vi "methane method.vi"(7 "pattern":string, 8 "error in (not an error)":errorcluster, 9 "data in":T1={"scaling kPa/volt"=1032.0, "module"=1, "data interval (s)"=1, "First channel Set 1"=0, "First channel Set 2"=0, "Sample Set 1"=["", "", "", "", "", "", "", "", "", "", "", "", "", "", "", " "], "Sample Set 2"=["", "", "", "", "", "", "", "", "", "", "", "", "", "", "", " "], "Samples Set 1"=0, "Samples Set2"=0, "history length"=1000, "number Tue"=[], "number Wed"=[]} {"history length" min=1; "data interval (s)" min=1; "module" min=1 step=1}, 10 "Action":enum16{"Save", "Open"}(ring)) -> (0 "error out":errorcluster, 1 "data out":T1={"scaling kPa/volt"=1032.0, "module"=1, "data interval (s)"=1, "First channel Set 1"=0, "First channel Set 2"=0, "Sample Set 1"=["", "", "", "", "", "", "", "", "", "", "", "", "", "", "", " "], "Sample Set 2"=["", "", "", "", "", "", "", "", "", "", "", "", "", "", "", " "], "Samples Set 1"=0, "Samples Set2"=0, "history length"=1000, "number Tue"=[], "number Wed"=[]} {"history length" min=1; "data interval (s)" min=1; "module" min=1 step=1})   [LabVIEW 2010]
uses:
  DAC apps/support/methane method.ctl
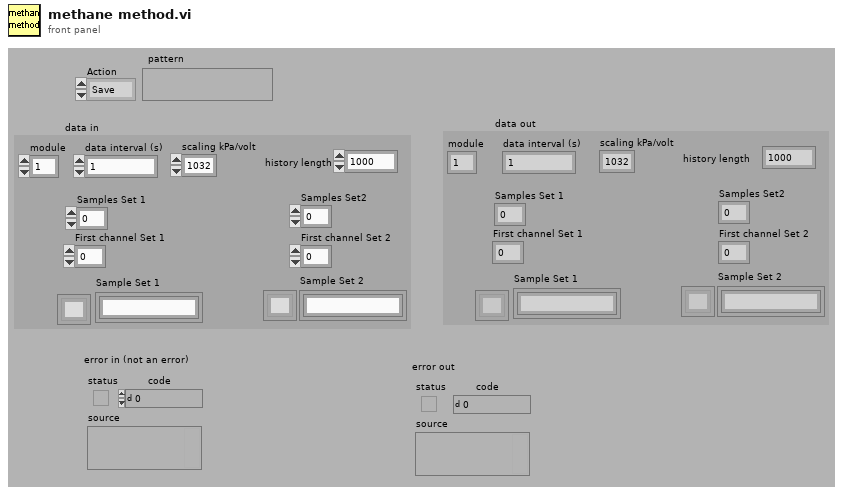
[diagram p1: front panel]
types:
  T1 = typedef "methane method.ctl" = cluster{"scaling kPa/volt":dbl, "module":u8, "data interval (s)":i32, "First channel Set 1":i8, "First channel Set 2":i8, "Sample Set 1":string[], "Sample Set 2":string[], "Samples Set 1":i8, "Samples Set2":i8, "history length":u16, "number Tue":string[], "number Wed":string[]}
  T2 = enum16{"open", "open or create", "create or replace", "create", "open (read only)"}
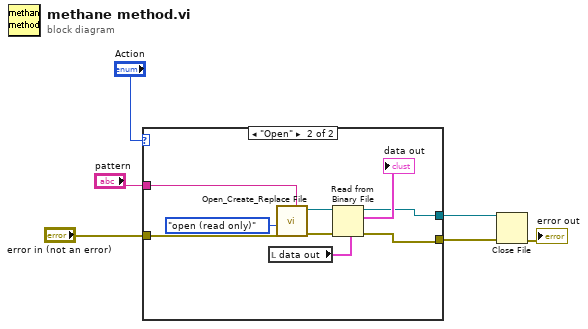
[diagram p0: block diagram]
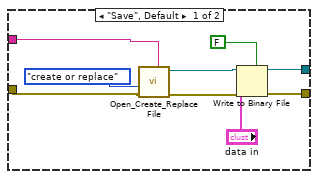
[diagram p2: hidden frame]
diagram:
  n1 = case shown="\"Open\"" "Action" {
    tunnel: [w9 w19] -> w6
    tunnel: [w10 w18] -> w5
    tunnel: "pattern" -> [w14 w23]
    tunnel: "error in (not an error)" -> [w13 w17]
    frame "Save", Default {
      n2 = call <vilib>:"Open_Create_Replace File.vi"("pattern"=w14, "error in (no error)"=w13, "function (open:0)"=T2."create or replace") -> ("error out"=w11:errorcluster, "refnum"=w12:refnum<file>)  [unwired: 5 in, 2 out]
      n3 = Write to Binary File(file (use dialog)=w12, data="data in", error in=w11, 5:FALSE ("prepend array or string size? (T)")) -> (refnum out=w9:refnum<file>, error out=w10:errorcluster)  [unwired: 2 in, 1 out]
    }
    frame "Open" {
      n4 = local read "data out"() -> (w16:T1)
      n5 = call <vilib>:"Open_Create_Replace File.vi"("pattern"=w23, "error in (no error)"=w17, "function (open:0)"=T2."open (read only)") -> ("error out"=w21:errorcluster, "refnum"=w22:refnum<file>)  [unwired: 5 in, 2 out]
      n6 = Read from Binary File(5:w16, 8:w21, 11:w22) -> (0:w18:errorcluster, 2:→"data out":T1, 3:w19:refnum<file>)  [unwired: 3 in, 1 out]
    }
  }
  n7 = Close File(refnum=w6, error in=w5) -> (error out=→"error out":errorcluster)  [unwired: 1 out]
